vi "SETPORT.vi"(8 "error in (no error)":errorcluster, 9 "Valor":string, 10 "Port":dbl, 11 "simulado in":refnum<class "simulado.lvclass">) -> (0 "error out":errorcluster, 3 "simulado out":refnum<class "simulado.lvclass">)   [LabVIEW 2019, in "simulado.lvclass"]
uses:
  simulado.lvclass
  simulado.lvclass/simulado.ctl
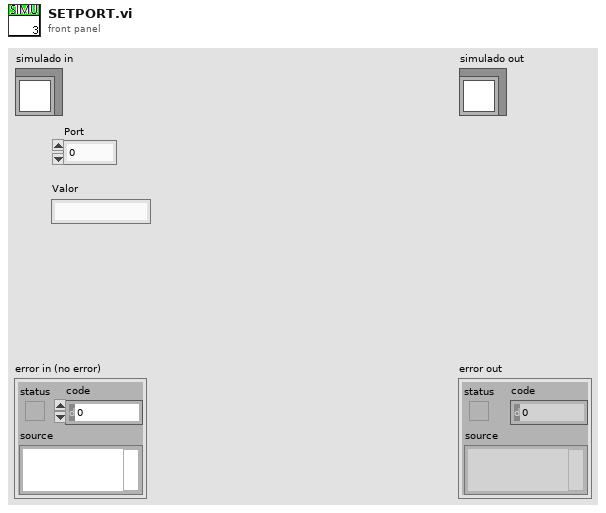
[diagram p1: front panel]
types:
  T1 = enum16{"get parameter", "Set parameters", "reset parameter", ""}
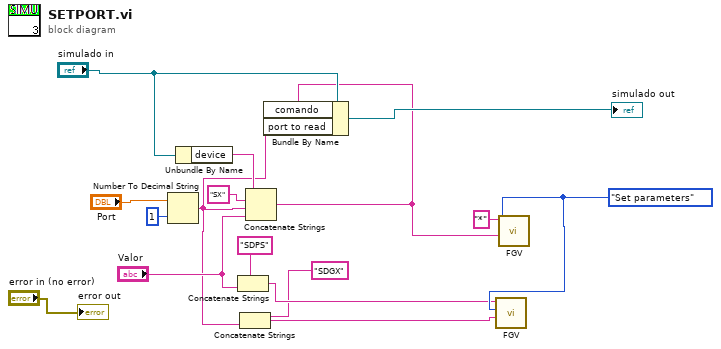
[diagram p0: block diagram]
diagram:
  w7 = T1."Set parameters" ("functions")
  n1 = Number To Decimal String(number="Port", width (-)=i16 1) -> (decimal integer string=w1:string)
  n2 = Unbundle By Name("simulado in") -> ("device"=w16:string)
  n3 = Concatenate Strings("SDPS" ("string"), "Valor") -> (w6:string)
  n4 = Concatenate Strings("SDGX" ("string"), w1) -> (w3:string)
  n5 = Concatenate Strings(w16, "SX" ("string"), w1, "Valor") -> (w10:string)
  n6 = Bundle By Name(cluster="simulado in", "comando"=w10, "port to read"=w1) -> (→"simulado out":refnum<class "simulado.lvclass">)
  n7 = call "FGV.vi"("command"=w3, "functions"=w7, "response to save"=w6) -> ()  [unwired: 7 in, 2 out]
  n8 = call "FGV.vi"("command"=w10, "functions"=w7, "response to save"="*") -> ()  [unwired: 7 in, 2 out]
  "error out" <- "error in (no error)"
